vi "MathCad_Matrix_Create.vi"(3 "error in (no error)":errorcluster, 5 "Worksheet Reference In":refnum<k7>) -> (0 "error out":errorcluster, 1 "Mathcad.IMatrixValue Reference Out":refnum<k7>, 2 "Worksheet Reference Out":refnum<k7>)   [LabVIEW 2015]
doc: "This creates a reference. A reference must be created before the value can be set and then inserted into the worksheet."
panel:
  in  "Mathcad.IMatrixValue Descriptor Type":refnum<k7>
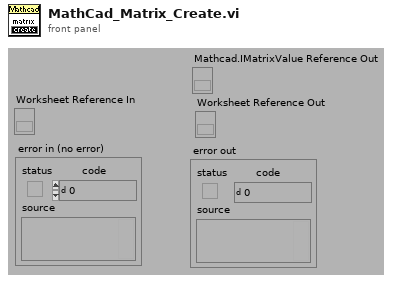
[diagram p1: front panel]
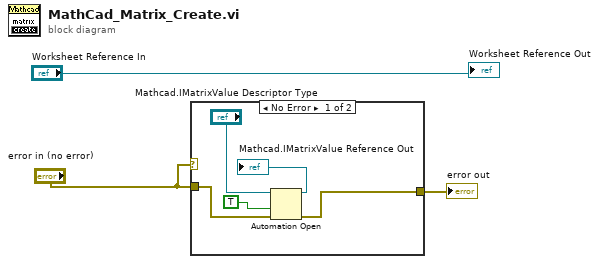
[diagram p0: block diagram]
diagram:
  n1 = case shown="No Error" "error in (no error)" {
    tunnel: "error in (no error)" -> [w6 w9]
    tunnel: [w5 w9] -> w2
    frame No Error {
      n2 = Automation Open(error in (no error)=w6, Automation Refnum="Mathcad.IMatrixValue Descriptor Type", 9:TRUE ("open new instance")) -> (Automation Refnum=→"Mathcad.IMatrixValue Reference Out":refnum<k7>, error out=w5:errorcluster)  [unwired: 1 in]
    }
    frame Error {
    }
  }
  "error out" <- w2
  "Worksheet Reference Out" <- "Worksheet Reference In"
